vi "Set Window Z-Position.vi"(8 "error in":errorcluster caption="error in (no error)" {"code" format="%d\n%x"}, 9 "No Activate? (T)":bool=TRUE, 10 "z-order position":u64(ring) items=["Not Topmost", "Topmost", "Top", "Bottom"], 11 "window refnum":T1) -> (0 "error out":errorcluster {"code" format="%d\n%x"}, 3 "window refnum out":T1)   [LabVIEW 2020, in "MacroAssert.lvlib" / "Win Util.lvlib"]
uses:
  Win Util.lvlib
  user32.dll
  Window Refnum.ctl
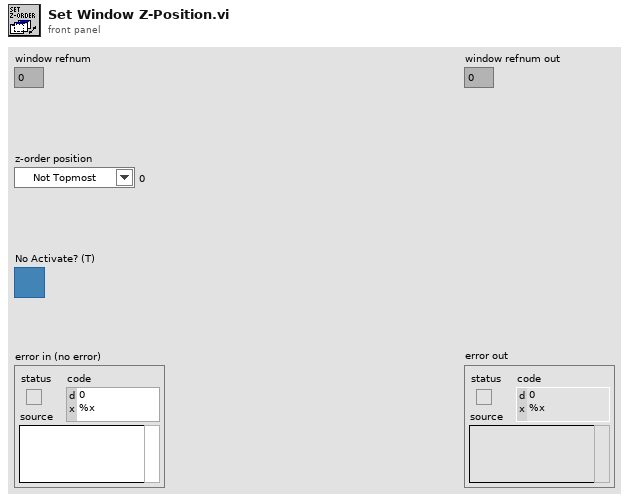
[diagram p1: front panel]
types:
  T1 = typedef "MacroAssert.lvlib/Win Util.lvlib/Window Refnum.ctl" = u64
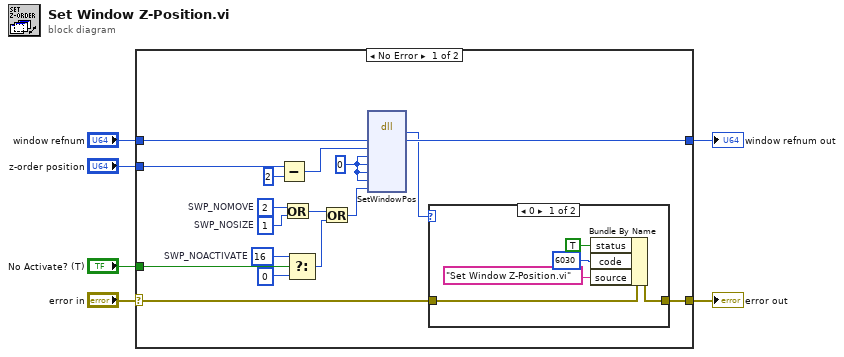
[diagram p0: block diagram]
diagram:
  n1 = case shown="No Error" "error in" {
    selector: "error in" -> [w14 w31]
    tunnel: [w15 w31] -> w6
    tunnel: [w10 w30] -> w5
    tunnel: "window refnum" -> [w13 w30]
    tunnel: "z-order position" -> [w12 _]
    tunnel: "No Activate? (T)" -> [w11 _]
    frame No Error {
      w18 = u32 2  # SWP_NOMOVE
      w19 = u32 1  # SWP_NOSIZE
      w8 = u32 16  # SWP_NOACTIVATE
      w23 = 0
      n2 = Subtract(x=w12, y=u64 2) -> (x-y=w17:u64)
      n3 = Or(x=w18, y=w19) -> (x .or. y?=w21:u32)
      n4 = Select(t=w8, s=w11, f=u32 0) -> (s? t:f=w20:u32)
      n5 = Or(x=w21, y=w20) -> (x .or. y?=w22:u32)
      n6 = dll-call lib="USER32.DLL" fn="SetWindowPos"("hWnd"=w13, "hWndInsertAfter"=w17, "left"=w23, "top"=w23, "width"=w23, "height"=w23, "fuFlags"=w22) -> ("error"=w9:i32, "hWnd"=w10:u64)  [unwired: 8 in, 3 out]
      n7 = case shown="0" w9 {
        tunnel: [w27 w29] -> w15
        tunnel: w14 -> [w26 w29]
        frame 0 {
          n8 = Bundle By Name(cluster=w26, "status"=TRUE, "code"=6030, "source"="Set Window Z-Position.vi") -> (w27:errorcluster)
        }
        frame Default {
        }
      }
    }
    frame Error {
    }
  }
  "window refnum out" <- w5
  "error out" <- w6
